vi "PM-sinal-modulation.vi"() -> ()   [LabVIEW 2013]
panel:
  in  "fm":dbl(slide) caption="Frequencia do sinal" min=0.0 max=10000.0 step=100.0 scale=0.0..10000.0
  in  "fp":dbl(slide) caption="Frequencia da portadora" min=0.0 max=10000.0 step=100.0 scale=0.0..10000.0
  in  "Kf":dbl(slide) caption="Constante de proporcionalidade (Kt)" min=0.0 max=10000.0 step=100.0 scale=0.0..100.0
  out "mod":cluster{dbl[], dbl[]}(graph) caption="Modulação"
  out "Portadora":cluster{dbl[], dbl[]}(graph)
  out "Informação":cluster{dbl[], dbl[]}(graph)
  in  "dt":dbl caption="Precisao temporal"
  in  "E0":dbl caption="Amplitude da portadora"
  in  "Em":dbl caption="Amplitude do sinal modulador"
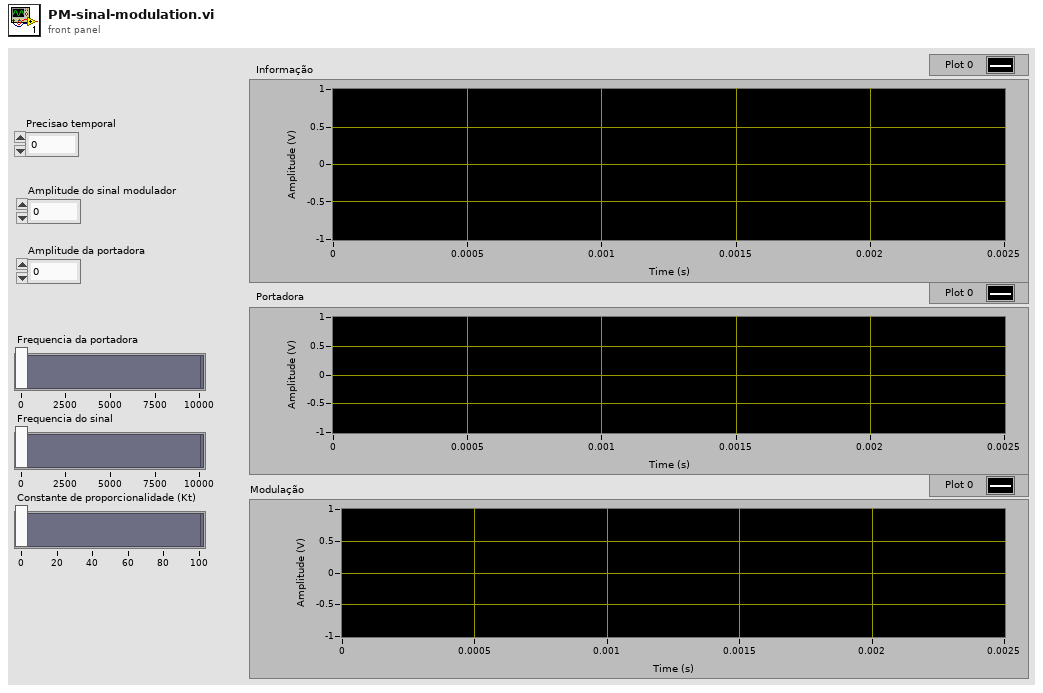
[diagram p1: front panel]
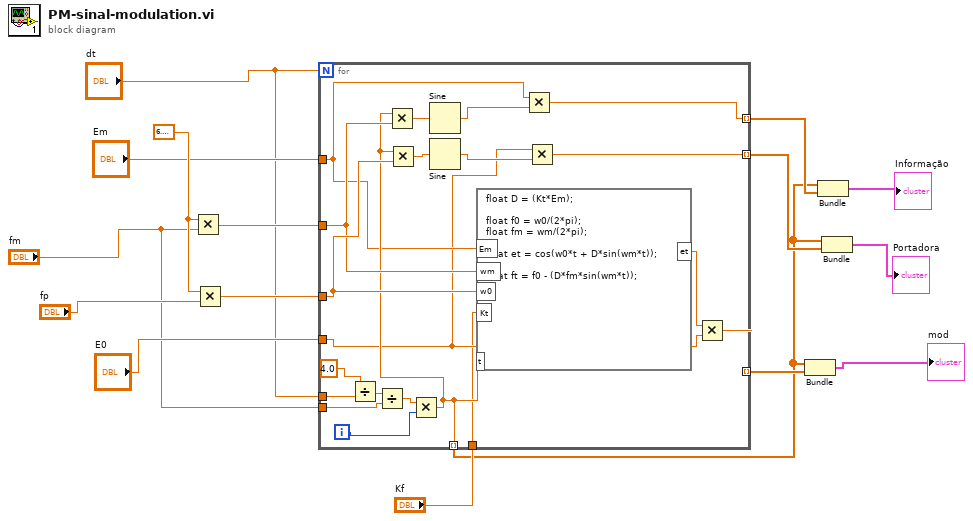
[diagram p0: block diagram]
diagram:
  w16 = 6.283185307179586
  n1 = Multiply(x=w16, y="fm") -> (x*y=w14:dbl)
  n2 = Multiply(x=w16, y="fp") -> (x*y=w15:dbl)
  n3 = for {
    N: "dt" -> [_]
    tunnel: "Em" -> [w21]
    tunnel: "E0" -> [w20]
    tunnel: w14 -> [w28]
    tunnel: w15 -> [w29]
    tunnel: "dt" -> [w36]
    tunnel: [w19] -> w10 mode=indexing
    tunnel: [w18] -> w9 mode=indexing
    tunnel: [w26] -> w6 mode=indexing
    tunnel: "Kf" -> [w17]
    tunnel: "fm" -> [w25]
    tunnel: [w24] -> w1 mode=indexing
    i -> [w32]
    n4 = Divide(x=4.0, y=w36) -> (x/y=w34:dbl)
    n5 = Divide(x=w34, y=w25) -> (x/y=w33:dbl)
    n6 = Multiply(x=w33, y=w32) -> (x*y=w24:dbl)
    n7 = Multiply(x=w24, y=w28) -> (x*y=w31:dbl)
    n8 = Multiply(x=w24, y=w29) -> (x*y=w30:dbl)
    n9 = Sine(x=w31) -> (sin(x)=w23:dbl)
    n10 = Sine(x=w30) -> (sin(x)=w22:dbl)
    n11 = formula code="float D = (Kt*Em);\n\nfloat f0 = w0/(2*pi);\nfloat fm = wm/(2*pi);\n\nfloat et = cos(w0*t + D*sin(wm*t));\n\nfloat ft = f0 - (D*fm*sin(wm*t));"("wm"=w28, "w0"=w29, "t"=w24, "Em"=w21, "Kt"=w17) -> ("et"=w27:dbl)
    n12 = Multiply(x=w21, y=w23) -> (x*y=w19:dbl)
    n13 = Multiply(x=w20, y=w22) -> (x*y=w18:dbl)
    n14 = Multiply(x=w27, y=w20) -> (x*y=w26:dbl)
  }
  n15 = Bundle(w1, w6) -> (→"mod":cluster{dbl[], dbl[]})  [unwired: 1 in]
  n16 = Bundle(w1, w10) -> (→"Informação":cluster{dbl[], dbl[]})  [unwired: 1 in]
  n17 = Bundle(w1, w9) -> (→"Portadora":cluster{dbl[], dbl[]})  [unwired: 1 in]
